vi "Write String Refnum.vi"(8 "error in (no error)":errorcluster, 10 "Ring Refnum":refnum<vi>, 11 "Ring Control in":refnum<class "Ring Control.lvclass">) -> (0 "error out":errorcluster, 3 "Ring Control out":refnum<class "Ring Control.lvclass">)   [LabVIEW 2010, in "Ring Control.lvclass"]
uses:
  Ring Control.lvclass
  Ring Control.lvclass/Ring Control.ctl
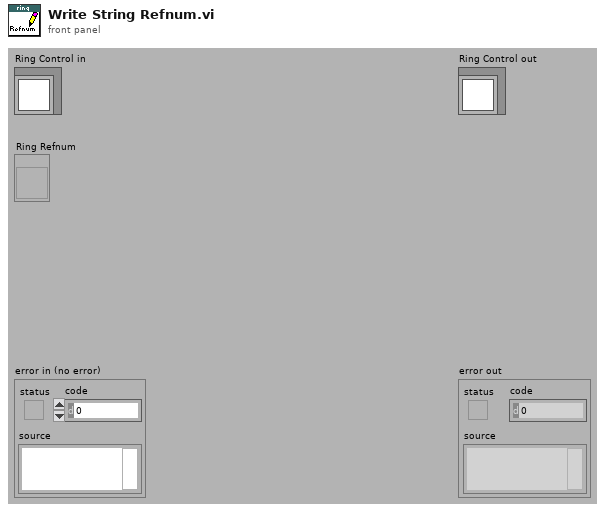
[diagram p1: front panel]
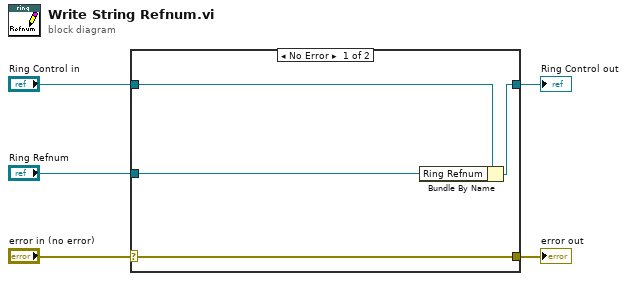
[diagram p0: block diagram]
diagram:
  n1 = case shown="No Error" "error in (no error)" {
    selector: "error in (no error)" -> [w9 w10]
    tunnel: [w9 w10] -> w4
    tunnel: [w7 w11] -> w2
    tunnel: "Ring Control in" -> [w8 w11]
    tunnel: "Ring Refnum" -> [w6 _]
    frame No Error {
      n2 = Bundle By Name(cluster=w8, "Ring Refnum"=w6) -> (w7:refnum<class "Ring Control.lvclass">)
    }
    frame Error {
    }
  }
  "error out" <- w4
  "Ring Control out" <- w2
